vi "CalculateXYZ.vi"(3 "CMF":dbl[][](array[numeric]), 4 "Reflectance":dbl[](array[numeric]), 5 "Illuminant":dbl[](array[numeric])) -> (0 "Z":dbl, 1 "Y":dbl, 2 "X":dbl)   [LabVIEW 2014]
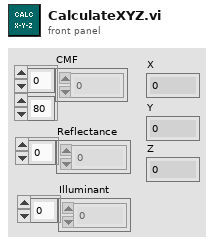
[diagram p1: front panel]
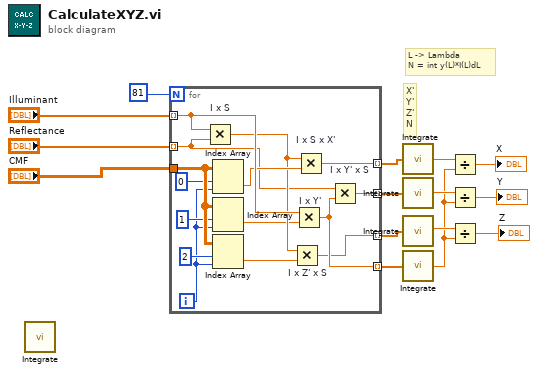
[diagram p0: block diagram]
diagram:
  # "X'\nY'\nZ'\nN"
  # "L -> Lambda\nN = int y(L)*I(L)dL"
  n1 = call "Integrate.vi"() -> ()  [unwired: 1 in, 1 out]
  n2 = for {
    N: 81 -> [_]
    tunnel: "CMF" -> [w30]
    tunnel: "Illuminant" -> [w29] mode=indexing
    tunnel: "Reflectance" -> [w25] mode=indexing
    tunnel: [w24] -> w1 mode=indexing
    tunnel: [w23] -> w3 mode=indexing
    tunnel: [w22] -> w4 mode=indexing
    tunnel: [w21] -> w2 mode=indexing
    i -> [w17]
    n3 = Multiply "I x S"(x=w29, y=w25) -> (x*y=w27:dbl)
    n4 = Index Array(array=w30, index (row)=0 ("disabled index (col)"), index (col)=w17) -> (element=w28:dbl)
    n5 = Index Array(array=w30, index (row)=1 ("disabled index (col)"), index (col)=w17) -> (element=w26:dbl)
    n6 = Index Array(array=w30, index (row)=2 ("disabled index (col)"), index (col)=w17) -> (element=w16:dbl)
    n7 = Multiply "I x Z' x S"(x=w27, y=w16) -> (x*y=w21:dbl)
    n8 = Multiply "I x Y'"(x=w29, y=w26) -> (x*y=w24:dbl)
    n9 = Multiply "I x S x X'"(x=w27, y=w28) -> (x*y=w22:dbl)
    n10 = Multiply "I x Y' x S"(x=w25, y=w24) -> (x*y=w23:dbl)
  }
  n11 = call "Integrate.vi"("Array"=w4) -> ("Integral result"=w14:dbl)
  n12 = call "Integrate.vi"("Array"=w3) -> ("Integral result"=w13:dbl)
  n13 = call "Integrate.vi"("Array"=w2) -> ("Integral result"=w12:dbl)
  n14 = call "Integrate.vi"("Array"=w1) -> ("Integral result"=w11:dbl)
  n15 = Divide(x=w14, y=w11) -> (x/y=→"X":dbl)
  n16 = Divide(x=w13, y=w11) -> (x/y=→"Y":dbl)
  n17 = Divide(x=w12, y=w11) -> (x/y=→"Z":dbl)
